vi "ANSI CRC16.vi"(11 "puchMsg":string) -> (1 "CRC校验":string, 2 "数据段":string, 3 "数据段长度":string)   [LabVIEW 2016]
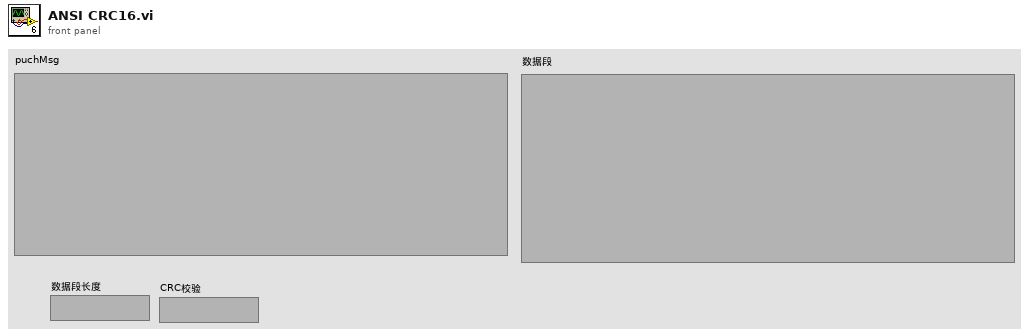
[diagram p1: front panel]
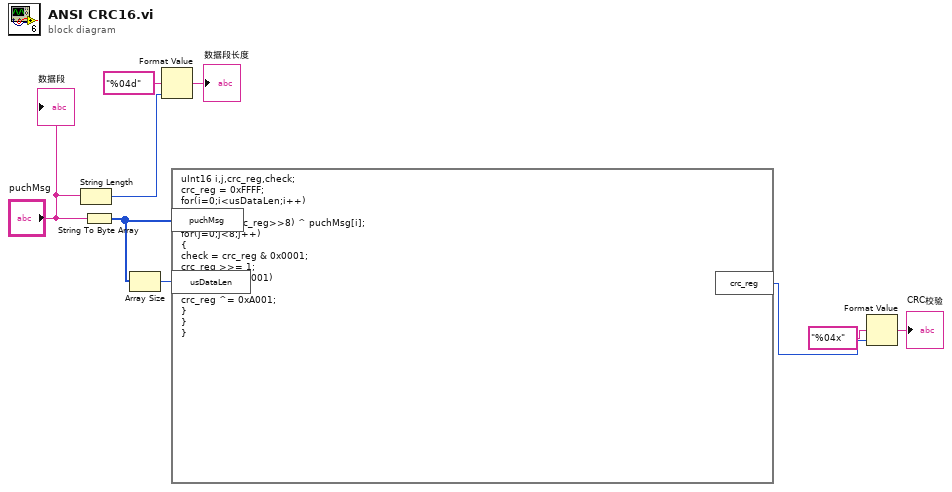
[diagram p0: block diagram]
diagram:
  n1 = String Length(string="puchMsg") -> (length=w7:i32)
  n2 = String To Byte Array(string="puchMsg") -> (unsigned byte array=w9:u8[])
  n3 = Array Size(array=w9) -> (size(s)=w8:i32)
  n4 = Format Value(format string="%04d" ("格式字符串"), value (0)=w7) -> (output string=→"数据段长度":string)  [unwired: 1 in]
  n5 = formula code="uInt16 i,j,crc_reg,check;\ncrc_reg = 0xFFFF;\nfor(i=0;i<usDataLen;i++)\n{\ncrc_reg = (crc_reg>>8) ^ puchMsg[i];\nfor(j=0;j<8;j++)\n{\ncheck = crc_reg & 0x0001;\ncrc_reg >>= 1;\nif(check==0x0001)\n{\ncrc_reg ^= 0xA001;\n}\n}\n}"("puchMsg"=w9, "usDataLen"=w8) -> ("crc_reg"=w2:u16)
  n6 = Format Value(format string="%04x" ("格式字符串"), value (0)=w2) -> (output string=→"CRC校验":string)  [unwired: 1 in]
  "数据段" <- "puchMsg"
